vi "Get header index.vi"(10 "key":string, 11 "header map in":map{string, i32}(c390)) -> (1 "found":bool, 2 "value out":i32, 3 "header map out":map{string, i32}(c390))   [LabVIEW 2020, in "Configuration_Helper.lvlib"]
uses:
  Configuration_Helper.lvlib
  <vilib>/Utility/miscctls.llb/LVMapReplaceAction.ctl
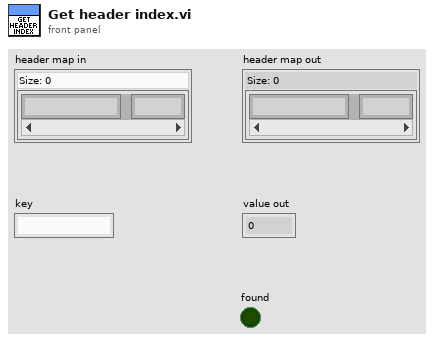
[diagram p1: front panel]
types:
  T1 = typedef "LVMapReplaceAction.ctl" = enum32{"Modify Entry only if found", "Add or Modify Entry", "Delete Entry"}
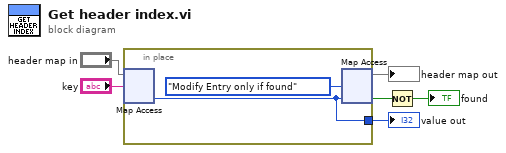
[diagram p0: block diagram]
diagram:
  n1 = in-place {
    in-place-border: [w7] -> w3
    n2 = in-place-map #1("header map in", "key") -> (w7:i32)  [unwired: 1 in, 1 out]
    n3 = in-place-map #1(w7, LVMapReplaceAction."Modify Entry only if found" ("action")) -> (→"header map out":map{string, i32}, w2:bool)  [unwired: 1 out]
  }
  "value out" <- w3
  n4 = Not(x=w2) -> (.not. x?=→"found":bool)
